vi "display.vi"(8 "error in (no error)":errorcluster caption="错误输入（无错误）", 11 "DGUS 输入":refnum<class "DGUS.lvclass">) -> (0 "error out":errorcluster caption="错误输出", 2 "字符串":string, 3 "DGUS 输出":refnum<class "DGUS.lvclass">)   [LabVIEW 2016, in "DGUS.lvlib" / "DGUS.lvclass"]
uses:
  DGUS.lvclass
  DGUS.lvclass/DGUS.ctl
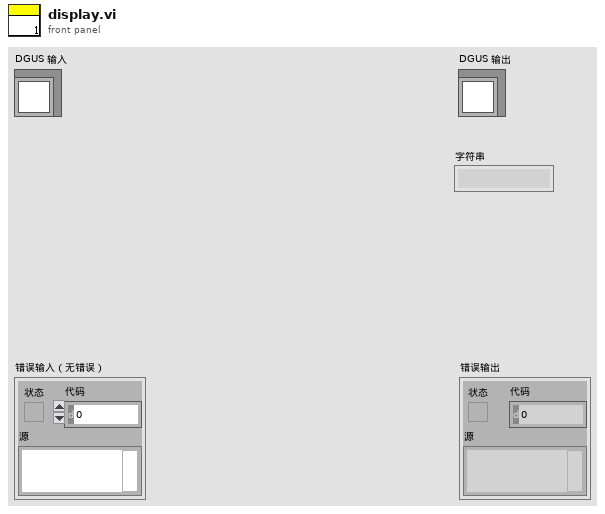
[diagram p1: front panel]
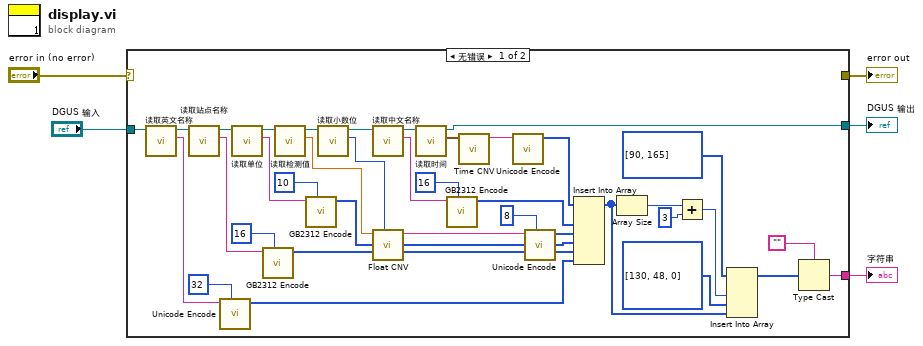
[diagram p0: block diagram]
diagram:
  n1 = case shown="无错误" "error in (no error)" {
    selector: "error in (no error)" -> [_ w44]
    tunnel: [_ w44] -> w4
    tunnel: [w31 w43] -> w2
    tunnel: "DGUS 输入" -> [w33 w43]
    tunnel: [w6 _] -> w1
    frame No Error {
      n2 = call "读取英文名称.vi"("DGUS输入"=w33) -> ("英文名称"=w34:string, "DGUS输出"=w16:refnum<class "DGUS.lvclass">)  [unwired: 8 in, 1 out]
      n3 = call "读取站点名称.vi"("DGUS输入"=w16) -> ("站点名称"=w35:string, "DGUS输出"=w20:refnum<class "DGUS.lvclass">)  [unwired: 8 in, 1 out]
      n4 = call "Unicode Encode.vi"("个数"=32, "字符串"=w34) -> ("数组"=w15:u8[])  [unwired: 9 in]
      n5 = call "读取单位.vi"("DGUS输入"=w20) -> ("单位"=w36:string, "DGUS输出"=w17:refnum<class "DGUS.lvclass">)  [unwired: 8 in, 1 out]
      n6 = call "GB2312 Encode.vi"("个数"=16, "字符串"=w35) -> ("数组"=w26:u8[])  [unwired: 9 in]
      n7 = call "读取检测值.vi"("DGUS输入"=w17) -> ("检测值"=w39:sgl, "DGUS输出"=w19:refnum<class "DGUS.lvclass">)  [unwired: 8 in, 1 out]
      n8 = call "GB2312 Encode.vi"("个数"=10, "字符串"=w36) -> ("数组"=w27:u8[])  [unwired: 9 in]
      n9 = call "读取小数位.vi"("DGUS输入"=w19) -> ("小数位"=w38:i16, "DGUS输出"=w18:refnum<class "DGUS.lvclass">)  [unwired: 8 in, 1 out]
      n10 = call "读取中文名称.vi"("DGUS输入"=w18) -> ("中文名称"=w40:string, "DGUS输出"=w32:refnum<class "DGUS.lvclass">)  [unwired: 8 in, 1 out]
      n11 = call "Float CNV.vi"("精度(6)"=w38, "数值"=w39) -> ("字符串"=w37:string)  [unwired: 9 in]
      n12 = call "读取时间.vi"("DGUS输入"=w32) -> ("时间"=w42:timestamp, "DGUS输出"=w31:refnum<class "DGUS.lvclass">)  [unwired: 8 in, 1 out]
      n13 = call "GB2312 Encode.vi"("个数"=16, "字符串"=w40) -> ("数组"=w29:u8[])  [unwired: 9 in]
      n14 = call "Time CNV.vi"("时间标识"=w42) -> ("字符串"=w41:string)  [unwired: 10 in]
      n15 = call "Unicode Encode.vi"("字符串"=w41) -> ("数组"=w30:u8[])  [unwired: 10 in]
      n16 = call "Unicode Encode.vi"("个数"=8, "字符串"=w37) -> ("数组"=w28:u8[])  [unwired: 9 in]
      n17 = Insert Into Array(array=w30, new element #1=w29, new element #2=w28, new element #3=w27, new element #4=w26, new element #5=w15) -> (w9:u8[])  [unwired: 1 in]
      n18 = Array Size(array=w9) -> (size(s)=w14:i32)
      n19 = Add(x=w14, y=3) -> (x+y=w11:i32)
      n20 = Insert Into Array(array=u8[] [90, 165] ("数组"), new element #1=w11, new element #2=u8[] [130, 48, 0] ("数组"), new element #3=w9) -> (w8:u8[])  [unwired: 1 in]
      n21 = Type Cast(type="", x=w8) -> (*(type *) &x=w6:string)
    }
    frame Error {
    }
  }
  "error out" <- w4
  "DGUS 输出" <- w2
  "字符串" <- w1
